vi "Status.vi"(7 "模式":enum16{"select", "insert", "update", "delete"}(ring), 10 "nameData":cluster{"name":string, "data":string}[](array[cluster])) -> (2 "元素":T1)   [LabVIEW 2013]
uses:
  <vilib>/addons/database/_DB Variant To Data/Database Variant To Data.xnode
panel:
  out "SQL query":string
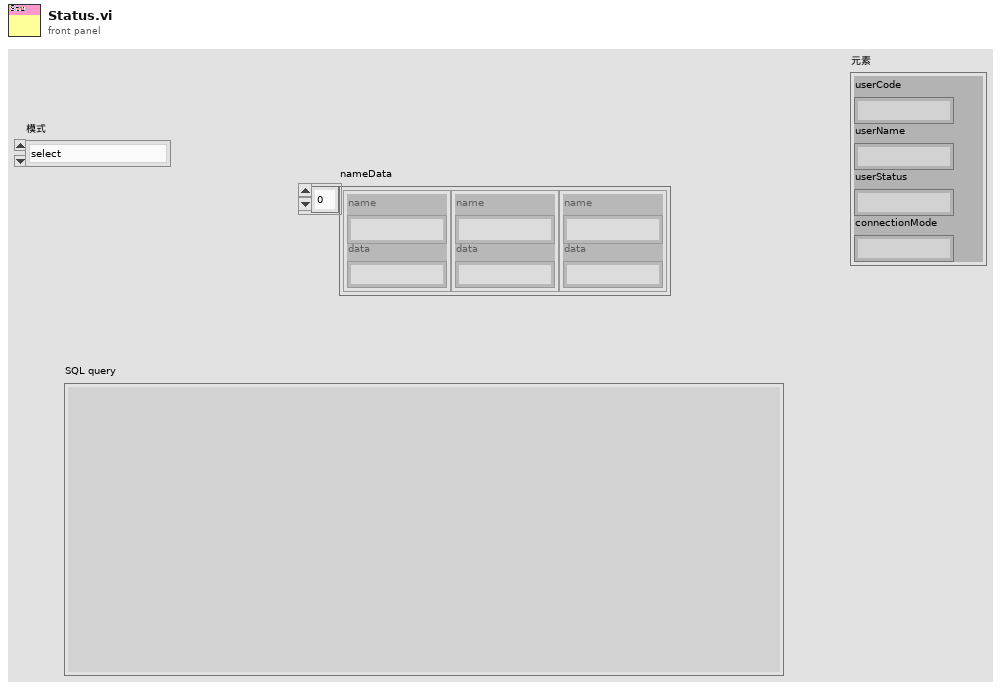
[diagram p1: front panel]
types:
  T1 = cluster{"userCode":string, "userName":string, "userStatus":string, "connectionMode":string}
  T2 = cluster{"CZZID":string, "CZZXM":string, "userStatus":string, "connectionMode":string}[]
  T3 = cluster{"CZZID":string, "CZZXM":string, "userStatus":string, "connectionMode":string}
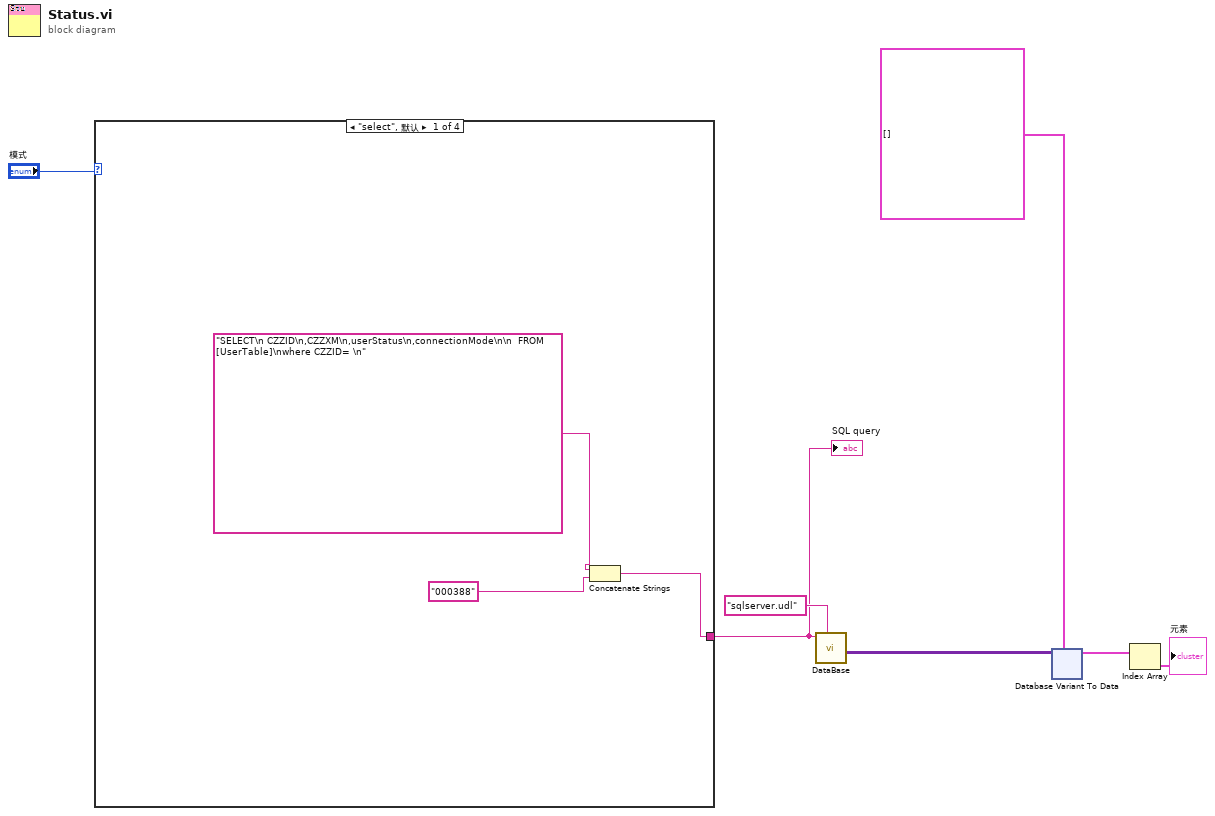
[diagram p0: block diagram]
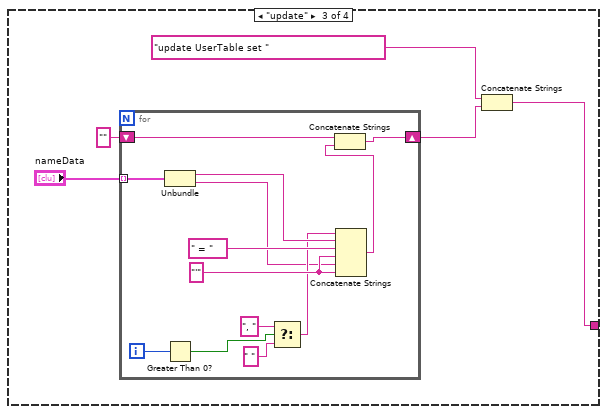
[diagram p3: hidden frame]
diagram:
  n1 = case shown="\"select\", 默认" "模式" {
    tunnel: [w8 _ w12 _] -> w4
    frame "select", Default {
      n2 = Concatenate Strings("SELECT\n CZZID\n,CZZXM\n,userStatus\n,connectionMode\n\n  FROM [UserTable]\nwhere CZZID= \n" ("SQL query"), "000388") -> (w8:string)
    }
    frame "insert" {
    }
    frame "update" {
      n3 = for {
        tunnel: "nameData" -> [w28] mode=indexing
        shift-right: [w26] -> w13
        shift-left: "" -> [w27]
        i -> [w25]
        w21 = "'" ("字符串")
        n4 = Unbundle(w28) -> ("name"=w19:string, "data"=w17:string)
        n5 = Greater Than 0?(x=w25) -> (x > 0?=w22:bool)
        n6 = Select(t=", " ("字符串"), s=w22, f=" " ("字符串")) -> (s? t:f=w18:string)
        n7 = Concatenate Strings(w18, w19, " = " ("SQL query"), w21, w17, w21) -> (w16:string)
        n8 = Concatenate Strings(w27, w16) -> (w26:string)
      }
      n9 = Concatenate Strings("update UserTable set " ("SQL query"), w13) -> (w12:string)
    }
    frame "delete" {
    }
  }
  "SQL query" <- w4
  n10 = call "DataBase.vi"("udl名称"="sqlserver.udl", "SQL query"=w4) -> ("recordset data"=w7:variant[][])  [unwired: 9 in]
  n11 = xnode ("Database Variant To Data")("database variant"=w7, "type"=T2 [] ("添加的数组")) -> ("data"=w2:T2)  [unwired: 1 in, 1 out]
  n12 = Index Array(array=w2) -> (element=→"元素":T3)  [unwired: 1 in]
